vi "Clear Task.vi"(8 "error in":errorcluster, 11 "Analog Output in":refnum<class "NI Analog Output.lvclass">) -> (0 "error out":errorcluster, 3 "Analog Output out":refnum<class "NI Analog Output.lvclass">)   [LabVIEW 2023, in "HardwareAbstractionLayer_LVOOP.lvlib" / "NI Analog Output.lvclass"]
doc: "DAQ AO Clear Data"
uses:
  NI Analog Output.lvclass
  NI Analog Output.lvclass/NI Analog Output.ctl
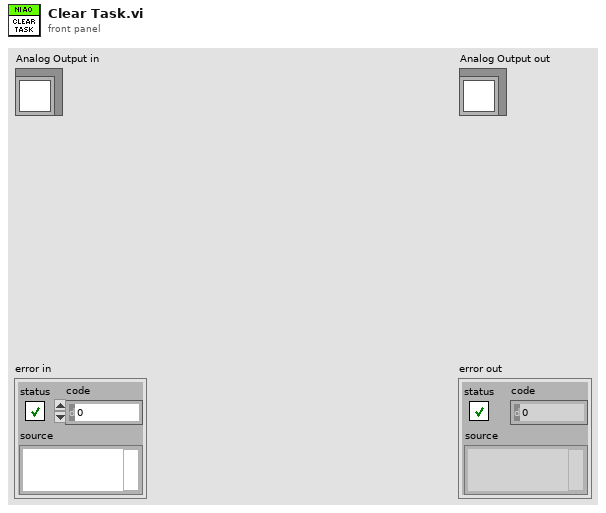
[diagram p1: front panel]
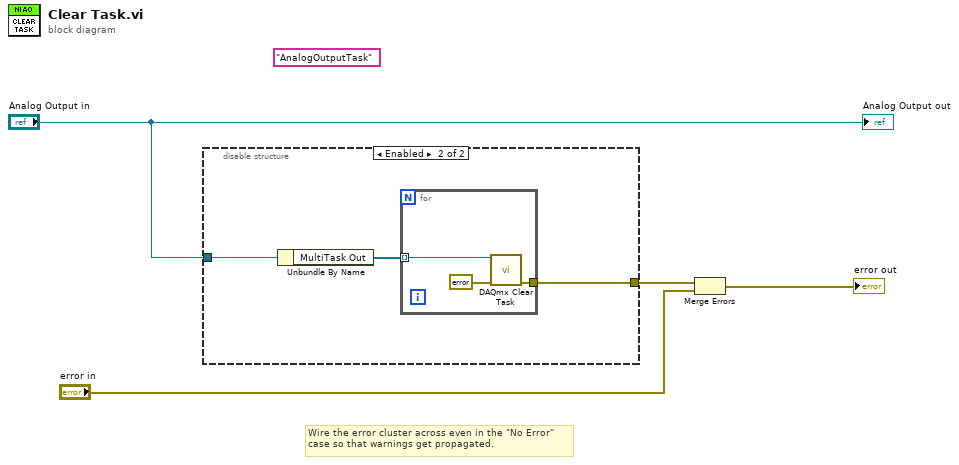
[diagram p0: block diagram]
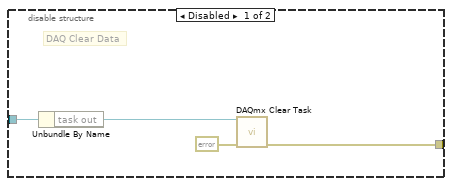
[diagram p2: hidden frame]
diagram:
  (unwired) "AnalogOutputTask" ("new task name")
  # "Wire the error cluster across even in the \"No Error\"\ncase so that warnings get propagated."
  n1 = disable-structure shown="Enabled" {
    disable-tunnel: [w8 w9] -> w4
    disable-tunnel: "Analog Output in" -> [w7 w10]
    frame Disabled {
      # "DAQ Clear Data"
      n2 = Unbundle By Name(w7) -> ("task out"=w6:refnum<k21>)
      n3 = call <vilib>:"DAQmx Clear Task.vi"("task in"=w6, "error in"=errorcluster {"status"=FALSE, "code"=0, "source"=""}) -> ("error out"=w8:errorcluster)  [unwired: 13 in]
    }
    frame Enabled {
      n4 = Unbundle By Name(w10) -> ("MultiTask Out"=w11:refnum<k21>[])
      n5 = for {
        tunnel: [w14] -> w9
        tunnel: w11 -> [w13] mode=indexing
        n6 = call <vilib>:"DAQmx Clear Task.vi"("task in"=w13, "error in"=errorcluster {"status"=FALSE, "code"=0, "source"=""}) -> ("error out"=w14:errorcluster)  [unwired: 13 in]
      }
    }
  }
  n7 = Merge Errors(w4, "error in") -> (→"error out":errorcluster)
  "Analog Output out" <- "Analog Output in"
